vi "外观 1.vi"(0 "Data In":T5=enum."采配水" caption="数据输入", 2 "Display State In":T3={"模块启用"={"电源管理禁用"=enum."Enabled", "采配水禁用"=enum."Enabled", "氨氮禁用"=enum."Enabled", "总磷总氮禁用"=enum."Enabled", "总氮禁用"=enum."Enabled", "多参数禁用"=enum."Enabled", "CODMn禁用"=enum."Enabled", "CODcr禁用"=enum."Enabled", "流量计禁用"=enum."Enabled", "质控单元禁用"=enum."Enabled", "超标留样禁用"=enum."Enabled", "其他禁用"=enum."Enabled"}, "模块名称"={"氨氮模块名称"="氨氮", "总磷总氮模块名称"="总磷总氮"}} caption="显示状态输入", 3 "Container State":T4 caption="容器状态") -> (6 "Data Out":T5=enum."采配水" caption="数据输出", 7 "Display State Out":T3={"模块启用"={"电源管理禁用"=enum."Enabled", "采配水禁用"=enum."Enabled", "氨氮禁用"=enum."Enabled", "总磷总氮禁用"=enum."Enabled", "总氮禁用"=enum."Enabled", "多参数禁用"=enum."Enabled", "CODMn禁用"=enum."Enabled", "CODcr禁用"=enum."Enabled", "流量计禁用"=enum."Enabled", "质控单元禁用"=enum."Enabled", "超标留样禁用"=enum."Enabled", "其他禁用"=enum."Enabled"}, "模块名称"={"氨氮模块名称"="氨氮", "总磷总氮模块名称"="总磷总氮"}} caption="显示状态输出", 8 "Action":T2 caption="动作")   [LabVIEW 2016, in "运维调试菜单.xctl"]
uses:
  <vilib>/_xctls/Container State.ctl
  <vilib>/_xctls/Action.ctl
  <vilib>/Utility/miscctls.llb/LVPointTypeDef.ctl
  <vilib>/_xctls/XControlSupport.lvlib
panel:
  in  "单选按钮":T1
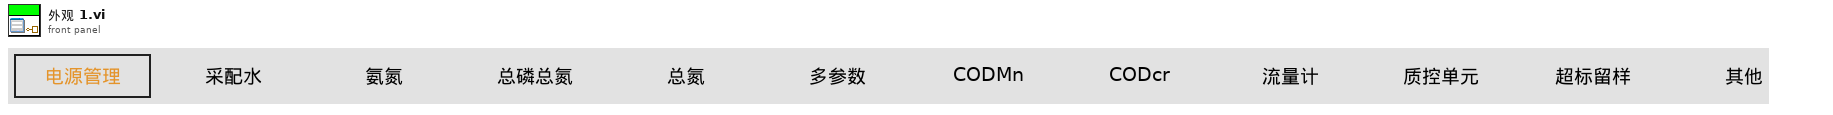
[diagram p1: front panel]
types:
  T1 = typedef "运维调试菜单.xctl/控件外观.ctl" = enum32{"电源管理", "采配水", "氨氮", "总磷总氮", "总氮", "多参数", "CODMn", "CODcr", "流量计", "质控单元", "超标留样", "其他"}
  T2 = typedef "XControlSupport.lvlib/Action.ctl" = cluster{"Data Changed?":bool, "State Changed?":bool, "Action Name":string}
  T3 = typedef "运维调试菜单.xctl/状态 1.ctl" = cluster{"模块启用":cluster{"电源管理禁用":enum16{"Enabled", "Disabled", "Disabled and Grayed Out"}, "采配水禁用":enum16{"Enabled", "Disabled", "Disabled and Grayed Out"}, "氨氮禁用":enum16{"Enabled", "Disabled", "Disabled and Grayed Out"}, "总磷总氮禁用":enum16{"Enabled", "Disabled", "Disabled and Grayed Out"}, "总氮禁用":enum16{"Enabled", "Disabled", "Disabled and Grayed Out"}, "多参数禁用":enum16{"Enabled", "Disabled", "Disabled and Grayed Out"}, "CODMn禁用":enum16{"Enabled", "Disabled", "Disabled and Grayed Out"}, "CODcr禁用":enum16{"Enabled", "Disabled", "Disabled and Grayed Out"}, "流量计禁用":enum16{"Enabled", "Disabled", "Disabled and Grayed Out"}, "质控单元禁用":enum16{"Enabled", "Disabled", "Disabled and Grayed Out"}, "超标留样禁用":enum16{"Enabled", "Disabled", "Disabled and Grayed Out"}, "其他禁用":enum16{"Enabled", "Disabled", "Disabled and Grayed Out"}}, "模块名称":cluster{"氨氮模块名称":string, "总磷总氮模块名称":string}}
  T4 = typedef "XControlSupport.lvlib/Container State.ctl" = cluster{"Indicator?":bool, "Run Mode?":bool, " Refnum":refnum<vi>}
  T5 = typedef "运维调试菜单.xctl/数据 1.ctl" = enum16{"电源管理", "采配水", "氨氮", "总磷总氮", "总氮", "多参数", "CODMn", "CODcr", "流量计", "质控单元", "超标留样", "其他"}
  T6 = typedef "LVPointTypeDef.ctl" = cluster{"Horizontal":i16, "Vertical":i16}
  T7 = cluster{"电源管理禁用":enum16{"Enabled", "Disabled", "Disabled and Grayed Out"}, "采配水禁用":enum16{"Enabled", "Disabled", "Disabled and Grayed Out"}, "氨氮禁用":enum16{"Enabled", "Disabled", "Disabled and Grayed Out"}, "总磷总氮禁用":enum16{"Enabled", "Disabled", "Disabled and Grayed Out"}, "总氮禁用":enum16{"Enabled", "Disabled", "Disabled and Grayed Out"}, "多参数禁用":enum16{"Enabled", "Disabled", "Disabled and Grayed Out"}, "CODMn禁用":enum16{"Enabled", "Disabled", "Disabled and Grayed Out"}, "CODcr禁用":enum16{"Enabled", "Disabled", "Disabled and Grayed Out"}, "流量计禁用":enum16{"Enabled", "Disabled", "Disabled and Grayed Out"}, "质控单元禁用":enum16{"Enabled", "Disabled", "Disabled and Grayed Out"}, "超标留样禁用":enum16{"Enabled", "Disabled", "Disabled and Grayed Out"}, "其他禁用":enum16{"Enabled", "Disabled", "Disabled and Grayed Out"}}
  T8 = enum16{"Enabled", "Disabled", "Disabled and Grayed Out"}[]
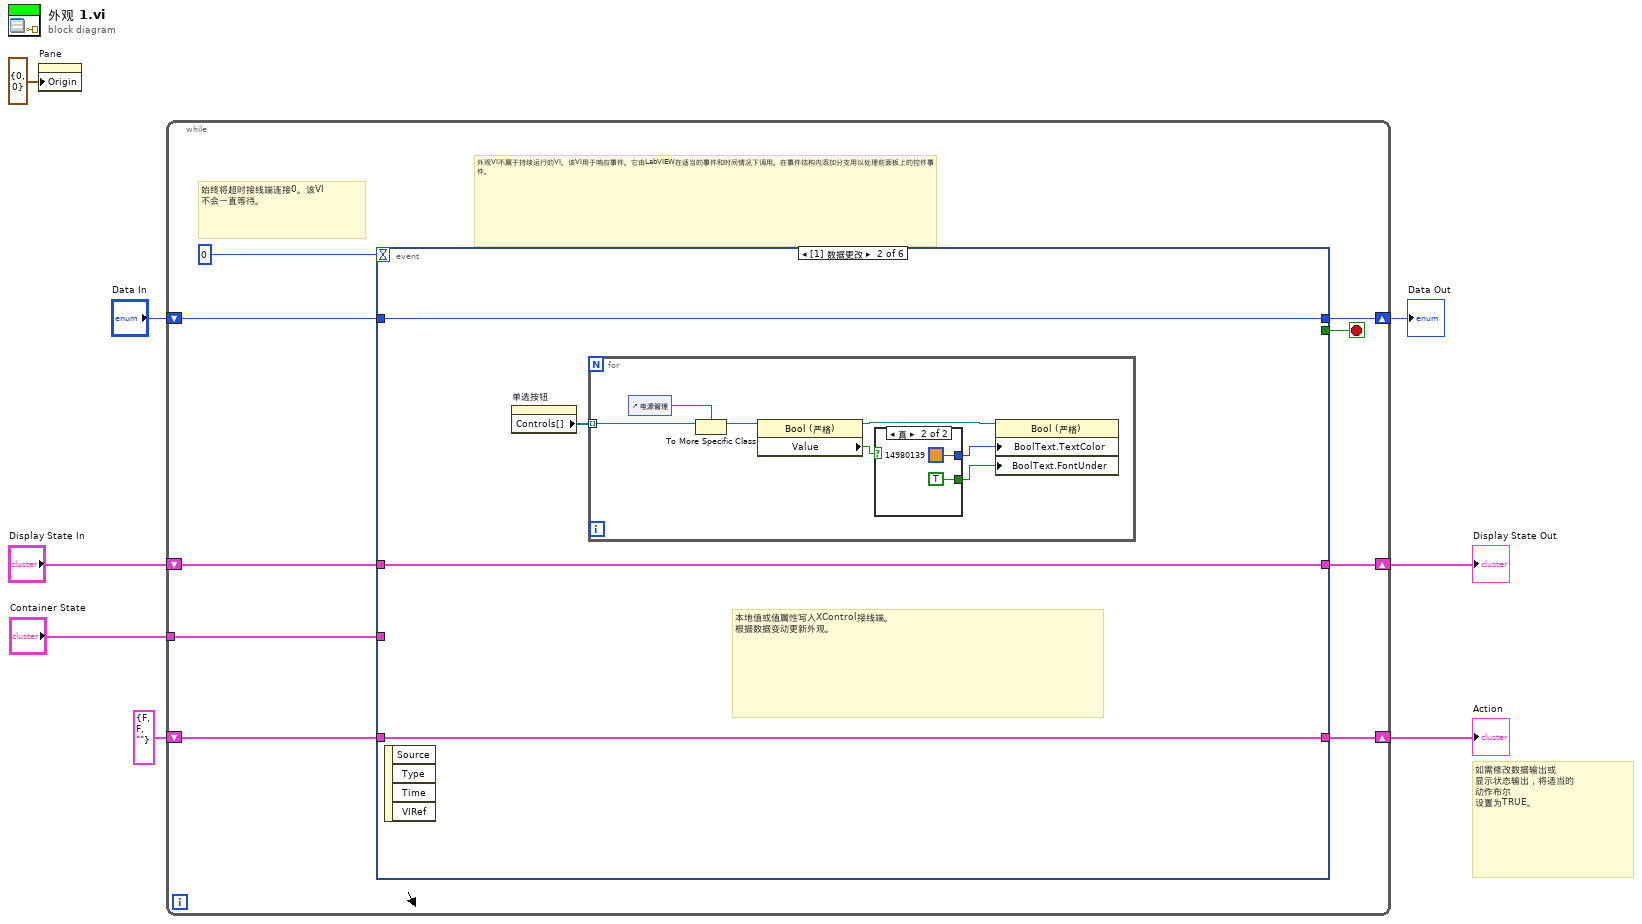
[diagram p0: block diagram]
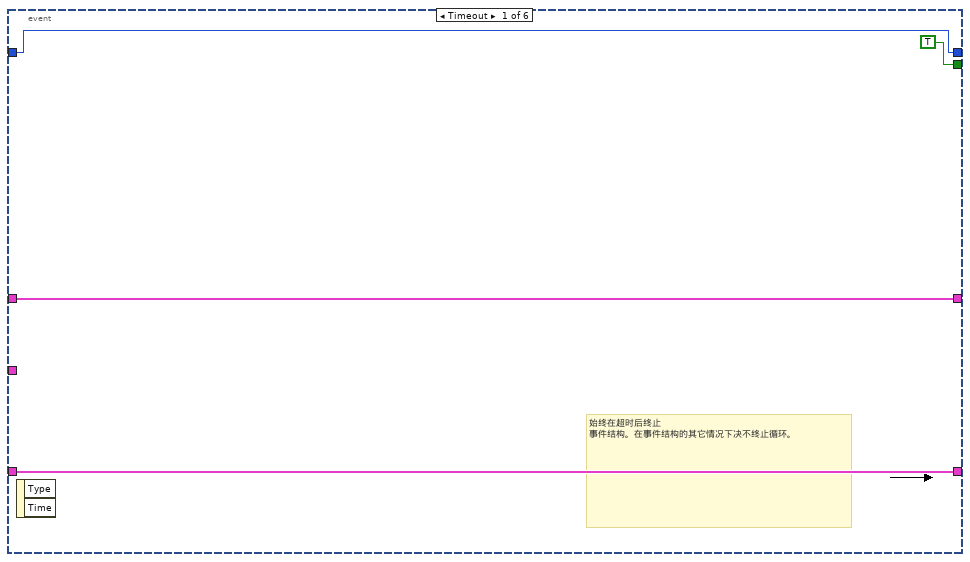
[diagram p2: hidden frame]
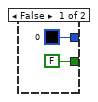
[diagram p3: hidden frame]
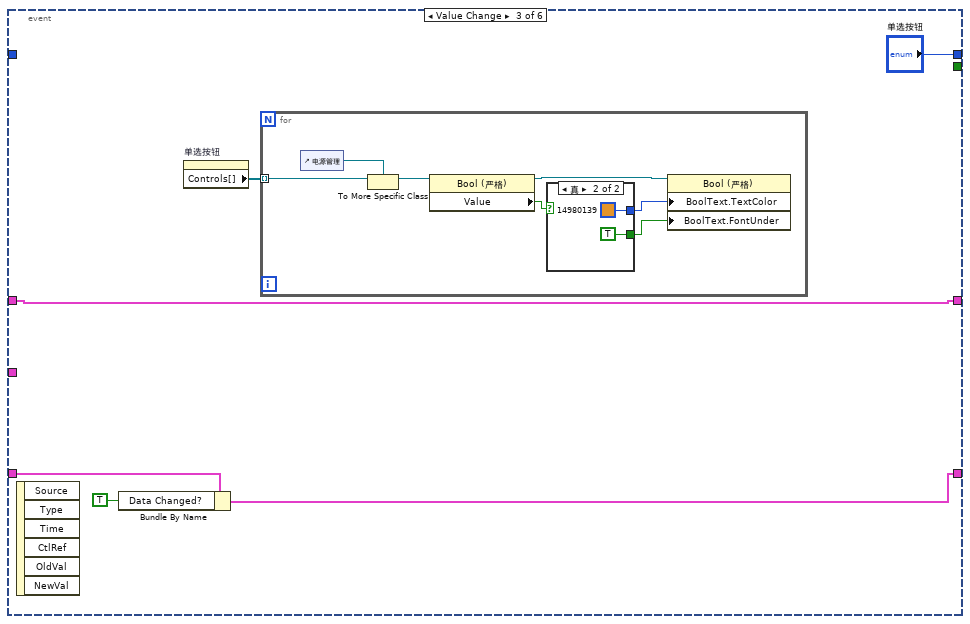
[diagram p4: hidden frame]
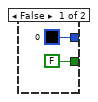
[diagram p5: hidden frame]
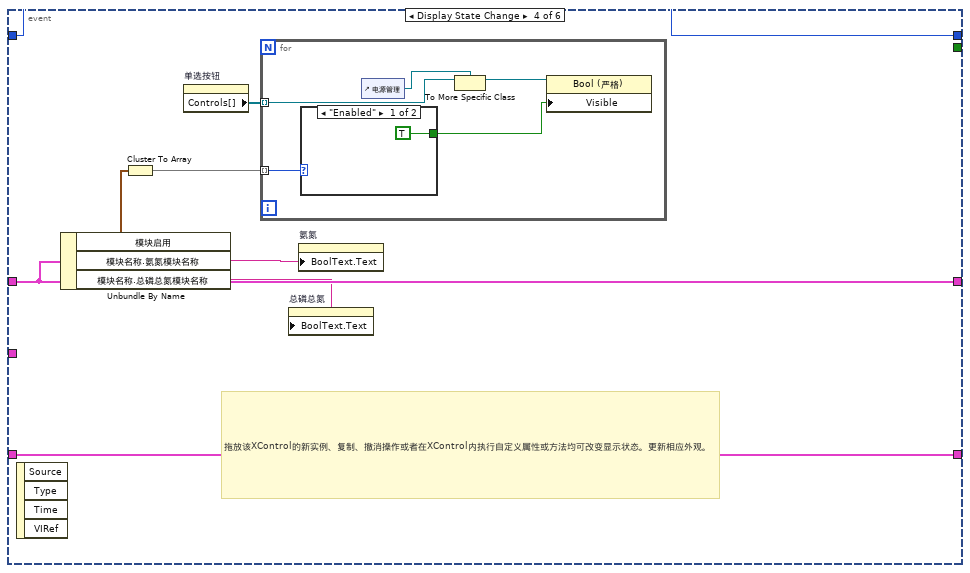
[diagram p6: hidden frame]
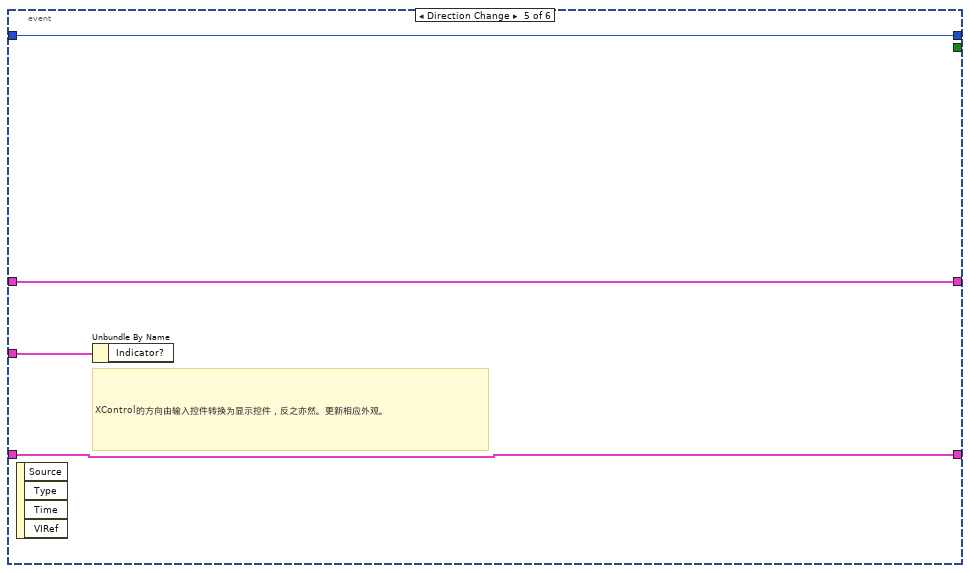
[diagram p8: hidden frame]
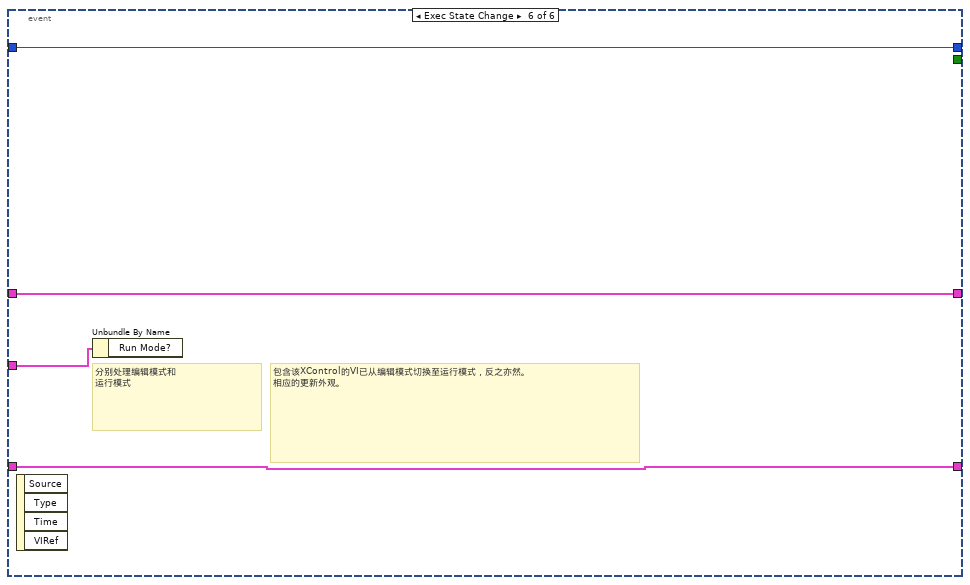
[diagram p9: hidden frame]
diagram:
  # "如需修改数据输出或\n显示状态输出，将适当的\n动作布尔\n设置为TRUE。"
  n1 = property on="Pane" class="Pane"("Origin"=T6 {"Horizontal"=0, "Vertical"=0} ("原点")) -> ()  [unwired: 2 in, 2 out]
  n2 = while {
    shift-right: [w16] -> w5
    shift-left: "Display State In" -> [w17]
    tunnel: "Container State" -> [w13]
    shift-right: [w11] -> w8
    shift-left: "Data In" -> [w12]
    shift-right: [w9] -> w3
    shift-left: T2 {"Data Changed?"=FALSE, "State Changed?"=FALSE, "Action Name"=""} ("Action") -> [w10]
    stop <- w15 stop-if-true
    # "外观VI不属于持续运行的VI。该VI用于响应事件。它由LabVIEW在适当的事件和时间情况下调用。在事件结构内添加分支用以处理前面板上的控件事件。"
    # "始终将超时接线端连接0。该VI\n不会一直等待。"
    n3 = event shown="[1] 数据更改" {
      selector: _ -> [_ _ _ _ _ _]
      dyn-events: _ -> [_ _ _ _ _ _]
      timeout: 0 -> [_ _ _ _ _ _]
      tunnel: w17 -> [w19 w24 w42 w57 w70 w74]
      tunnel: [w19 w24 w42 w57 w70 w74] -> w16
      tunnel: [TRUE _ _ _ _ _] -> w15
      tunnel: w13 -> [_ _ _ _ w71 w75]
      tunnel: w12 -> [w18 w25 _ w61 w69 w73]
      tunnel: [w18 w25 "单选按钮" w61 w69 w73] -> w11
      tunnel: [w20 w23 w40 w60 w68 w72] -> w9
      tunnel: w10 -> [w20 w23 w41 w60 w68 w72]
      event Timeout {
        # "始终在超时后终止\n事件结构。在事件结构的其它情况下决不终止循环。"
        n4 = event-data() -> ()  [unwired: 1 in, 2 out]
      }
      event Data Change {
        # "本地值或值属性写入XControl接线端。\n根据数据变动更新外观。"
        n5 = event-data() -> ()  [unwired: 1 in, 4 out]
        n6 = property on="单选按钮" class="RadioBtnsControl (严格)"() -> ("Controls[]"=w22:refnum<vi>[])  [unwired: 2 in, 2 out]
        n7 = for {
          tunnel: w22 -> [w32] mode=indexing
          n8 = control-ref of="电源管理"() -> (w31:refnum<vi>)
          n9 = To More Specific Class(target class=w31, reference=w32) -> (specific class reference=w30:refnum<vi>)  [unwired: 1 in, 1 out]
          n10 = property class="Bool (严格)"(reference=w30) -> (reference out=w29:refnum<vi>, "Value"=w28:bool)  [unwired: 1 in, 1 out]
          n11 = case shown="真" w28 {
            tunnel: [u32 0 u32 14980139] -> w27
            tunnel: [FALSE ("布尔文本.字体:下划线") TRUE ("布尔文本.字体:下划线")] -> w26
            frame False {
            }
            frame True {
            }
          }
          n12 = property class="Bool (严格)"(reference=w29, "BoolText.TextColor"=w27, "BoolText.FontUnder"=w26) -> ()  [unwired: 1 in, 2 out]
        }
      }
      event Value Change {
        n13 = event-data() -> ()  [unwired: 1 in, 6 out]
        n14 = Bundle By Name(cluster=w41, "Data Changed?"=TRUE) -> (w40:T2)
        n15 = property on="单选按钮" class="RadioBtnsControl (严格)"() -> ("Controls[]"=w37:refnum<vi>[])  [unwired: 2 in, 2 out]
        n16 = for {
          tunnel: w37 -> [w49] mode=indexing
          n17 = control-ref of="电源管理"() -> (w48:refnum<vi>)
          n18 = To More Specific Class(target class=w48, reference=w49) -> (specific class reference=w47:refnum<vi>)  [unwired: 1 in, 1 out]
          n19 = property class="Bool (严格)"(reference=w47) -> (reference out=w46:refnum<vi>, "Value"=w45:bool)  [unwired: 1 in, 1 out]
          n20 = case shown="真" w45 {
            tunnel: [u32 0 u32 14980139] -> w44
            tunnel: [FALSE ("布尔文本.字体:下划线") TRUE ("布尔文本.字体:下划线")] -> w43
            frame False {
            }
            frame True {
            }
          }
          n21 = property class="Bool (严格)"(reference=w46, "BoolText.TextColor"=w44, "BoolText.FontUnder"=w43) -> ()  [unwired: 1 in, 2 out]
        }
      }
      event Display State Change {
        # "拖放该XControl的新实例、复制、撤消操作或者在XControl内执行自定义属性或方法均可改变显示状态。更新相应外观。"
        n22 = event-data() -> ()  [unwired: 1 in, 4 out]
        n23 = Unbundle By Name(w57) -> ("模块启用"=w56:T7, "模块名称.氨氮模块名称"=w55:string, "模块名称.总磷总氮模块名称"=w54:string)
        n24 = Cluster To Array(cluster=w56) -> (array=w58:T8)
        n25 = property on="单选按钮" class="RadioBtnsControl (严格)"() -> ("Controls[]"=w59:refnum<vi>[])  [unwired: 2 in, 2 out]
        n26 = for {
          tunnel: w59 -> [w66] mode=indexing
          tunnel: w58 -> [w63] mode=indexing
          n27 = case shown="\"Enabled\"" w63 {
            tunnel: [TRUE ("布尔文本.字体:下划线") _] -> w62
            frame "Enabled" {
            }
            frame "Disabled", Default {
            }
          }
          n28 = control-ref of="电源管理"() -> (w65:refnum<vi>)
          n29 = To More Specific Class(target class=w65, reference=w66) -> (specific class reference=w64:refnum<vi>)  [unwired: 1 in, 1 out]
          n30 = property class="Bool (严格)"(reference=w64, "Visible"=w62) -> ()  [unwired: 1 in, 2 out]
        }
        n31 = property on="总磷总氮" class="Bool (严格)"("BoolText.Text"=w54) -> ()  [unwired: 2 in, 2 out]
        n32 = property on="氨氮" class="Bool (严格)"("BoolText.Text"=w55) -> ()  [unwired: 2 in, 2 out]
      }
      event Direction Change {
        # "XControl的方向由输入控件转换为显示控件，反之亦然。更新相应外观。"
        n33 = event-data() -> ()  [unwired: 1 in, 4 out]
        n34 = Unbundle By Name(w71) -> ()  [unwired: 1 out]
      }
      event Exec State Change {
        # "包含该XControl的VI已从编辑模式切换至运行模式，反之亦然。\n相应的更新外观。"
        # "分别处理编辑模式和\n运行模式"
        n35 = event-data() -> ()  [unwired: 1 in, 4 out]
        n36 = Unbundle By Name(w75) -> ()  [unwired: 1 out]
      }
    }
  }
  "Display State Out" <- w5
  "Data Out" <- w8
  "Action" <- w3
